vi "Calculate Desired States.vi"(8 "error in (no error)":errorcluster, 10 "Vessel In":refnum<class "Vessel.lvclass">, 11 "CJ Constant Jerk Guidance in":refnum<class "Constant Jerk Guidance.lvclass">) -> (0 "error out":errorcluster, 2 "Vessel Out":refnum<class "Vessel.lvclass">, 3 "CJ Constant Jerk Guidance out":refnum<class "Constant Jerk Guidance.lvclass">)   [LabVIEW 2014, in "Guidance Library.lvlib" / "Constant Jerk Guidance.lvclass"]
uses:
  Constant Jerk Guidance.lvclass
  ROV/Vessel.lvclass
  Library/Helping Routines/Rad 2 PI-PI Scalar.vi
  Library/Helping Routines/get_set_point (SubVI).vi
  Supervisor/Supervisor.lvclass
panel:
  in  "r_off":dbl[](array[numeric])=[0.5, 0.5, 0.0]
  out "Use Altitude Guidance":bool
  out "javr":dbl[](array[numeric])
  out "javp":dbl[](array[numeric])
  in  "jav rad 2":dbl[](array[numeric])=[0.15, 0.15, 0.25]
  in  "jav pos 2":dbl[](array[numeric])=[0.2, 0.2, 0.3]
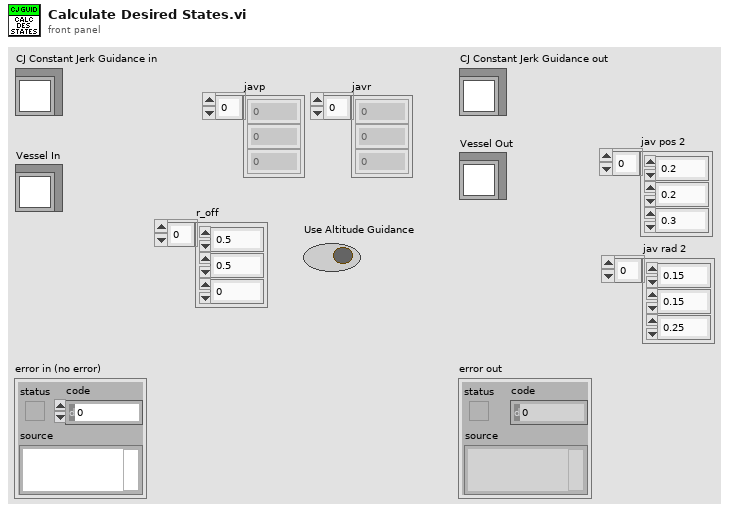
[diagram p1: front panel]
types:
  T1 = cluster{"Measured":cluster{"Eta":dbl[], "Nu":dbl[], "Eta Dot":dbl[], "Nu Dot":dbl[]}, "Estimated":cluster{"Eta":dbl[], "Nu":dbl[], "Eta Dot":dbl[], "Nu Dot":dbl[]}, "Desired":cluster{"Eta":dbl[], "Nu":dbl[], "Eta Dot":dbl[], "Nu Dot":dbl[]}, "Previous Desired":cluster{"Eta":dbl[], "Nu":dbl[], "Eta Dot":dbl[], "Nu Dot":dbl[]}, "tau":dbl[], "Altitude":cluster{"Measured":dbl, "Estimated":dbl, "Desired":dbl, "Previous Desired":dbl, "Approximated":dbl, "grad F":dbl[]}, "rpm":dbl[], "Attitude":cluster{"Theta Measured":dbl[], "Theta Estimated":dbl[], "Omega Measured":dbl[], "Omega Estimated":dbl[], "Gyro Bias":dbl[]}}
  T2 = cluster{"javp":dbl[], " javr":dbl[], "Break":bool, "arrived":bool, "arrived yaw":bool}
  T3 = cluster{"Set Origin":bool, "New WP":bool, "Types of Change":enum16{"Current NED", "Change NED"}, "Make Change":bool, "Optimal Heading":bool, "New SetPoint":cluster{"North":dbl, "East":dbl, "Depth":dbl, "Heading":dbl}, "Update Reference":cluster{"Mode Change":bool, "Current Position":dbl[]}, "Go":bool, "Go heading":bool}
  T4 = cluster{"North":dbl, "East":dbl, "Depth":dbl, "Heading":dbl}
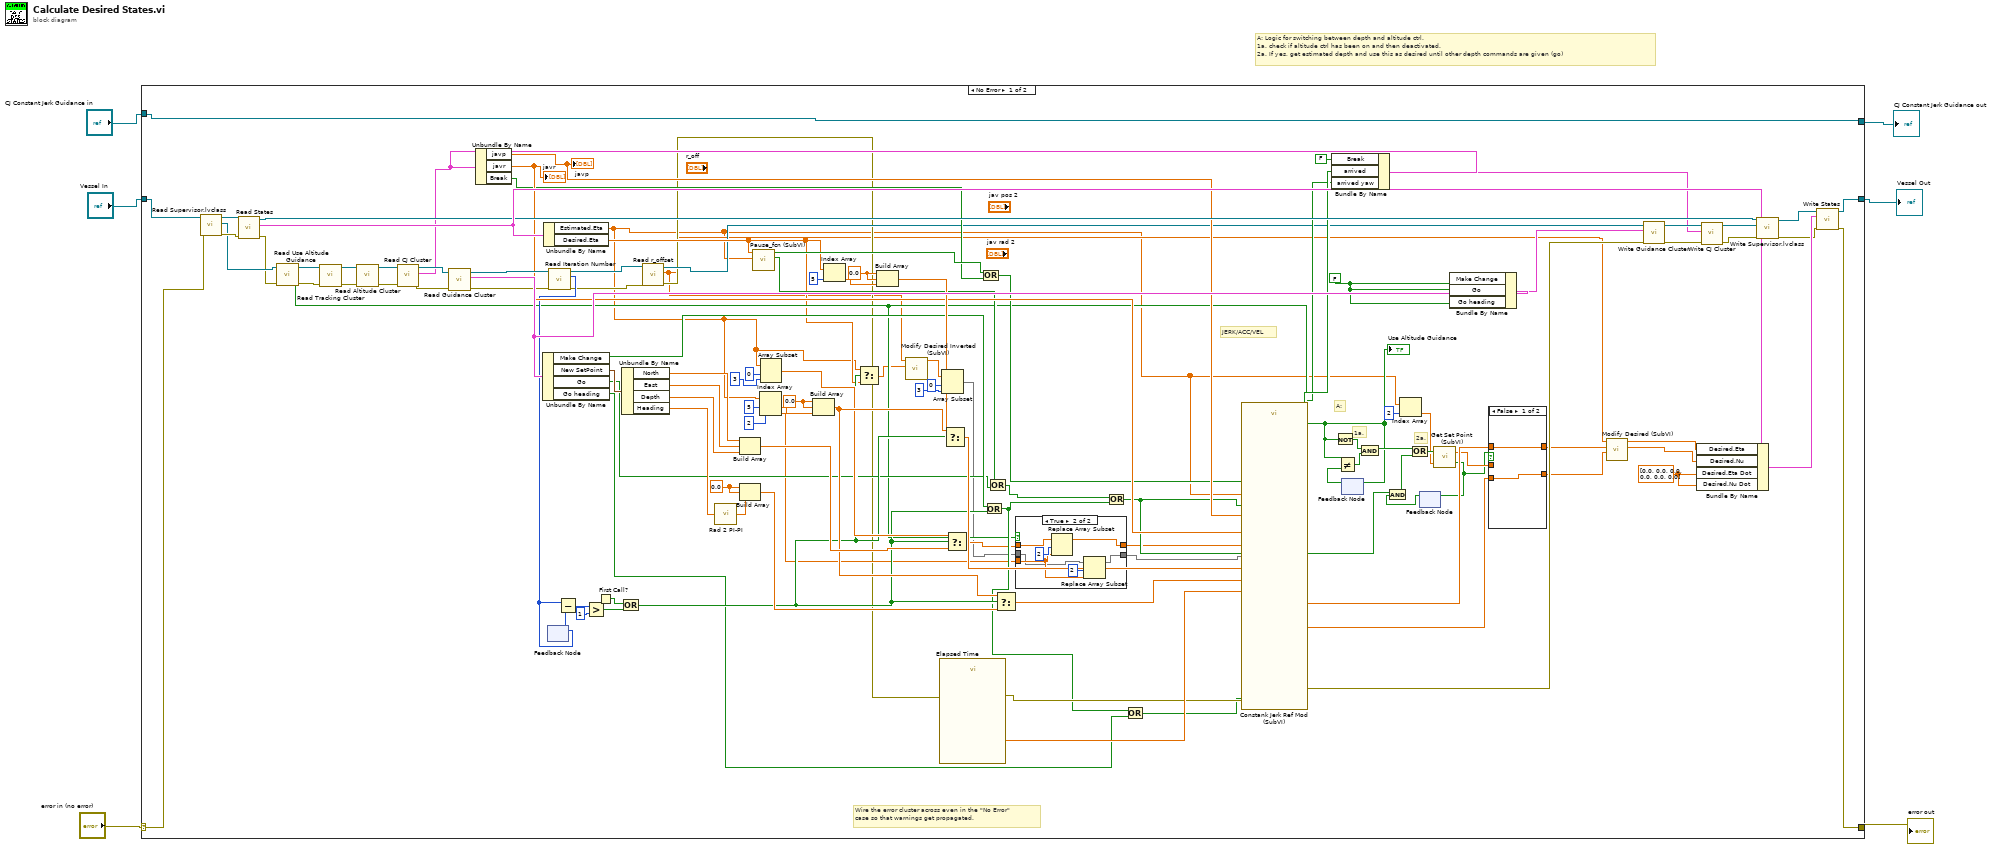
[diagram p0: block diagram]
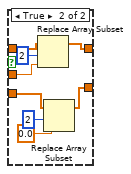
[diagram p3: hidden frame]
diagram:
  # "A: Logic for switching between depth and altitude ctrl. \n1a. check if altitude ctrl has been on and then deactivated.\n2a. If yes, get estimated depth and use this as desired until other depth commands are given (go)"
  n1 = case shown="No Error" "error in (no error)" {
    selector: "error in (no error)" -> [w105 w145]
    tunnel: [w95 w145] -> w5
    tunnel: "Vessel In" -> [w119 w143]
    tunnel: [w123 w143] -> w3
    tunnel: "CJ Constant Jerk Guidance in" -> [w59 w144]
    tunnel: [w59 w144] -> w1
    frame No Error {
      w72 = 0.0 ("element")
      w55 = FALSE ("Make Change")
      w109 = 0.0 ("element")
      w113 = 0.0 ("element")
      w120 = dbl[] [0.0, 0.0, 0.0, 0.0, 0.0, 0.0] ("Desired.Eta Dot")
      # "JERK/ACC/VEL"
      # "2a."
      # "1a."
      # "A:"
      # "Wire the error cluster across even in the \"No Error\"\ncase so that warnings get propagated."
      n2 = call "Read Supervisor.lvclass.vi"("error in (no error)"=w105, "Vessel in"=w119) -> ("error out"=w85:errorcluster, "Supervisor.lvclass"=w44:refnum<class "Supervisor.lvclass">, "Vessel out"=w118:refnum<class "Vessel.lvclass">)  [unwired: 7 in]
      n3 = call-dynamic "Read States.vi"("error in (no error)"=w85, "Vessel in"=w118) -> ("error out"=w42:errorcluster, "States"=w122:T1, "Vessel out"=w99:refnum<class "Vessel.lvclass">)  [unwired: 7 in]
      n4 = call-dynamic "Read Use Altitude Guidance.vi"("error in (no error)"=w42, "Supervisor in"=w44) -> ("error out"=w41:errorcluster, "Use Altitude Guidance"=w26:bool, "Supervisor out"=w43:refnum<class "Supervisor.lvclass">)  [unwired: 7 in]
      "Use Altitude Guidance" <- w26
      n5 = call-dynamic "Read Tracking Cluster.vi"("error in (no error)"=w41, "Supervisor in"=w43) -> ("error out"=w47:errorcluster, "Supervisor out"=w48:refnum<class "Supervisor.lvclass">)  [unwired: 7 in, 1 out]
      n6 = call-dynamic "Read Altitude Cluster.vi"("error in (no error)"=w47, "Supervisor in"=w48) -> ("error out"=w45:errorcluster, "Supervisor out"=w46:refnum<class "Supervisor.lvclass">)  [unwired: 7 in, 1 out]
      n7 = call-dynamic "Read CJ Cluster.vi"("error in (no error)"=w45, "Supervisor in"=w46) -> ("error out"=w83:errorcluster, "CJ Cluster"=w82:T2, "Supervisor out"=w84:refnum<class "Supervisor.lvclass">)  [unwired: 7 in]
      n8 = call-dynamic "Read Guidance Cluster.vi"("error in (no error)"=w83, "Supervisor in"=w84) -> ("error out"=w93:errorcluster, "Guidance Cluster"=w101:T3, "Supervisor out"=w94:refnum<class "Supervisor.lvclass">)  [unwired: 7 in]
      n9 = Unbundle By Name(w82) -> ("javp"=w65:dbl[], "javr"=w64:dbl[], "Break"=w53:bool)
      "javp" <- w65
      "javr" <- w64
      n10 = Unbundle By Name(w101) -> ("Make Change"=w60:bool, "New SetPoint"=w117:T4, "Go"=w51:bool, "Go heading"=w58:bool)
      n11 = Unbundle By Name(w122) -> ("Estimated.Eta"=w7:dbl[], "Desired.Eta"=w17:dbl[])
      n12 = feedback #1() -> (w92:i32)  [unwired: 1 in]
      n13 = call-dynamic "Read Iteration Number.vi"("error in (no error)"=w93, "Supervisor in"=w94) -> ("error out"=w11:errorcluster, "Iteration Number"=w61:i32, "Supervisor out"=w13:refnum<class "Supervisor.lvclass">)  [unwired: 7 in]
      n14 = feedback-in #1(w61) -> ()
      n15 = Subtract(x=w61, y=w92) -> (x-y=w91:i32)
      n16 = Greater?(x=w91, y=1) -> (0:w89:bool)
      n17 = First Call?() -> (First Call?: T/F=w88:bool)
      n18 = Or(x=w88, y=w89) -> (x .or. y?=w66:bool)
      n19 = Unbundle By Name(w117) -> ("North"=w116:dbl, "East"=w115:dbl, "Depth"=w114:dbl, "Heading"=w87:dbl)
      n20 = call-dynamic "Read r_offset.vi"("error in (no error)"=w11, "Supervisor in"=w13) -> ("error out"=w10:errorcluster, "r_offset"=w9:dbl[], "Supervisor out"=w12:refnum<class "Supervisor.lvclass">)  [unwired: 7 in]
      n21 = call-poly "Rad 2 PI-PI.vi"("Angle In (rad)"=w87) -> ("Angle Out (pi-pi)"=w86:dbl)
      n22 = Build Array(w116, w115, w114) -> (w104:dbl[])
      n23 = Build Array(w113, w113, w86) -> (w103:dbl[])
      n24 = call "Pause_fcn (SubVI).vi"("Eta"=w7, "Eta_des"=w17) -> ("Go"=w50:bool, "Pause"=w54:bool)  [unwired: 8 in]
      n25 = Index Array(array=w7, index #1=5 ("index"), index #2=2 ("index")) -> (element #1=w108:dbl, element #2=w22:dbl)
      n26 = Array Subset(array=w7, index=0, length=3) -> (w67:dbl[])
      n27 = Build Array(w109, w109, w108) -> (w70:dbl[])
      n28 = Index Array(array=w17, index=5) -> (element=w73:dbl)
      n29 = Select(t=w7, s=w66, f=w17) -> (s? t:f=w16:dbl[])
      n30 = Build Array(w72, w72, w73) -> (w69:dbl[])
      n31 = call "Modify Desired Inverted (SubVI).vi"("Eta des"=w16, "r_off"=w9) -> ("eta_des_m"=w15:dbl[])  [unwired: 8 in, 1 out]
      n32 = call "Elapsed Time"("error in (no error)"=w10) -> ("Elapsed Time (s)"=w107:dbl, "error out"=w106:errorcluster)  [unwired: 11 in, 6 out]
      n33 = Array Subset(array=w15, index=0, length=3) -> (w14:dbl[])
      n34 = Select(t=w70, s=w66, f=w69) -> (s? t:f=w68:dbl[])
      n35 = Select(t=w67, s=w66, f=w104) -> (s? t:f=w24:dbl[])
      n36 = Or(x=w54, y=w53) -> (x .or. y?=w52:bool)
      n37 = Or(x=w60, y=w66) -> (x .or. y?=w56:bool)
      n38 = Or(x=w50, y=w51) -> (x .or. y?=w49:bool)
      n39 = Select(t=w70, s=w66, f=w103) -> (s? t:f=w102:dbl[])
      n40 = case shown="True" w26 {
        tunnel: w14 -> [w125 w127]
        tunnel: [w125 w129] -> w25
        tunnel: w24 -> [w124 w132]
        tunnel: [w124 w126] -> w8
        tunnel: w22 -> [_ w128]
        frame False {
        }
        frame True {
          n41 = Replace Array Subset(array=w132, new element=w128, index=2) -> (w126:dbl[])
          n42 = Replace Array Subset(array=w127, new element=w128, index=2) -> (w129:dbl[])
        }
      }
      n43 = Or(x=w49, y=w56) -> (x .or. y?=w36:bool)
      n44 = Or(x=w56, y=w58) -> (x .or. y?=w57:bool)
      n45 = call "Constank Jerk Ref Mod (SubVI).vi"("jav pos"=w65, "p_new"=w8, "Set point p"=w25, "Eta"=w7, "jav rad"=w64, "error in"=w106, "Brake"=w52, "Set point theta"=w68, "Go"=w36, "Go heading"=w57, "Theta_new"=w102, "time"=w107) -> ("Eta des"=w31:dbl[], "Arrived"=w63:bool, "Arrived yaw"=w62:bool, "Nu des"=w30:dbl[], "error out"=w97:errorcluster)  [unwired: 7 in, 4 out]
      n46 = Bundle By Name(cluster=w82, "Break"=FALSE, "arrived"=w63, "arrived yaw"=w62) -> (w76:T2)
      n47 = Not(x=w26) -> (.not. x?=w38:bool)
      n48 = feedback-in #2(w26) -> ()
      n49 = feedback #2() -> (w40:bool)  [unwired: 1 in]
      n50 = Not Equal?(x=w26, y=w40) -> (x != y?=w39:bool)
      n51 = And(x=w38, y=w39) -> (x .and. y?=w35:bool)
      n52 = Index Array(array=w7, index=2) -> (element=w32:dbl)
      n53 = feedback #3() -> (w37:bool)  [unwired: 1 in]
      n54 = And(x=w36, y=w37) -> (x .and. y?=w27:bool)
      n55 = Or(x=w35, y=w27) -> (x .or. y?=w34:bool)
      n56 = call-poly "Get Set Point (SubVI).vi"("set point in"=w32, "auto set  in"=w34) -> ("auto set"=w28:bool, "set point"=w29:dbl)
      n57 = feedback-in #3(w28) -> ()
      n58 = Bundle By Name(cluster=w101, "Make Change"=w55, "Go"=w55, "Go heading"=w55) -> (w100:T3)
      n59 = case shown="False" w28 {
        tunnel: w31 -> [w134 w142]
        tunnel: [w134 w135] -> w20
        tunnel: w30 -> [w133 w138]
        tunnel: [w133 w136] -> w19
        tunnel: w29 -> [_ w140]
        frame False {
        }
        frame True {
          n60 = Replace Array Subset(array=w142, new element=w140, index=2) -> (w135:dbl[])
          n61 = Replace Array Subset(array=w138, new element=0.0 ("new element/subarray"), index=2) -> (w136:dbl[])
        }
      }
      n62 = call "Modify Desired (SubVI).vi"("Nu des"=w19, "Eta des"=w20, "r_off"=w9) -> ("nu_des_m"=w18:dbl[], "eta_des_m"=w21:dbl[])  [unwired: 7 in]
      n63 = call-dynamic "Write Guidance Cluster.vi"("error in (no error)"=w97, "Guidance Cluster"=w100, "Supervisor in"=w12) -> ("error out"=w80:errorcluster, "Supervisor out"=w78:refnum<class "Supervisor.lvclass">)  [unwired: 7 in]
      n64 = Bundle By Name(cluster=w122, "Desired.Eta"=w21, "Desired.Nu"=w18, "Desired.Eta Dot"=w120, "Desired.Nu Dot"=w120) -> (w121:T1)
      n65 = call-dynamic "Write CJ Cluster.vi"("error in (no error)"=w80, "CJ Cluster"=w76, "Supervisor in"=w78) -> ("error out"=w79:errorcluster, "Supervisor out"=w77:refnum<class "Supervisor.lvclass">)  [unwired: 7 in]
      n66 = call "Write Supervisor.lvclass.vi"("error in (no error)"=w79, "Supervisor.lvclass"=w77, "Vessel in"=w99) -> ("error out"=w96:errorcluster, "Vessel out"=w98:refnum<class "Vessel.lvclass">)  [unwired: 7 in]
      n67 = call-dynamic "Write States.vi"("error in (no error)"=w96, "States"=w121, "Vessel in"=w98) -> ("error out"=w95:errorcluster, "Vessel out"=w123:refnum<class "Vessel.lvclass">)  [unwired: 7 in]
    }
    frame Error {
    }
  }
  "error out" <- w5
  "CJ Constant Jerk Guidance out" <- w1
  "Vessel Out" <- w3
